vi "SamplingAndSavingDlg.vi"(11 "采样过程中...in":u8(slide) scale=0.0..300.0) -> ()   [LabVIEW 2014, in "Sample.lvlib"]
uses:
  Sample/Sample.lvlib
panel:
  out "采样过程中...":u8(slide) scale=0.0..300.0
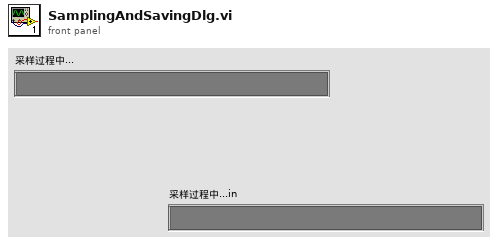
[diagram p1: front panel]
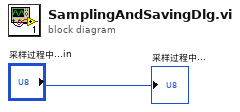
[diagram p0: block diagram]
diagram:
  "采样过程中..." <- "采样过程中...in"
